vi "pacmate.vi"() -> ()   [LabVIEW 2016]
uses:
  <vilib>/userdefined/High Color/IMAQdx.ctl
  <vilib>/vision/driver/NI_Vision_Acquisition_Software.lvlib
  <vilib>/vision/NI_Vision_Development_Module.lvlib
panel:
  out "filteredDiameter":dbl
  in  "LPF":dbl
  out "Numeric 2":dbl
  out "Numeric":dbl
  out "myDiameter":dbl
  out "Pos. X":i32
  in  "Low Thresh":i32
  in  "Mid Thresh":i32
  out "Min Radius":sgl
  in  "maxThresh":i32
  out "Radius":i32
  in  "Max Radius":sgl=10.0 format="%.2f"
  out "Circles Data":T1(array[cluster])
  out "Nb Circles":i32
  out "Image 3":T2(plugin-control)
  out "Image 2":T2(plugin-control)
  in  "Blue or Luma or Val or Inten Range":cluster{"Lower value":i32, "Upper value":i32}={"Lower value"=0, "Upper value"=255}
  in  "Green or Sat Range":cluster{"Lower value":i32, "Upper value":i32}={"Lower value"=0, "Upper value"=255}
  in  "Red or Hue Range":cluster{"Lower value":i32, "Upper value":i32}={"Lower value"=0, "Upper value"=255}
  out "Image":T2(plugin-control)
  in  "stop":bool
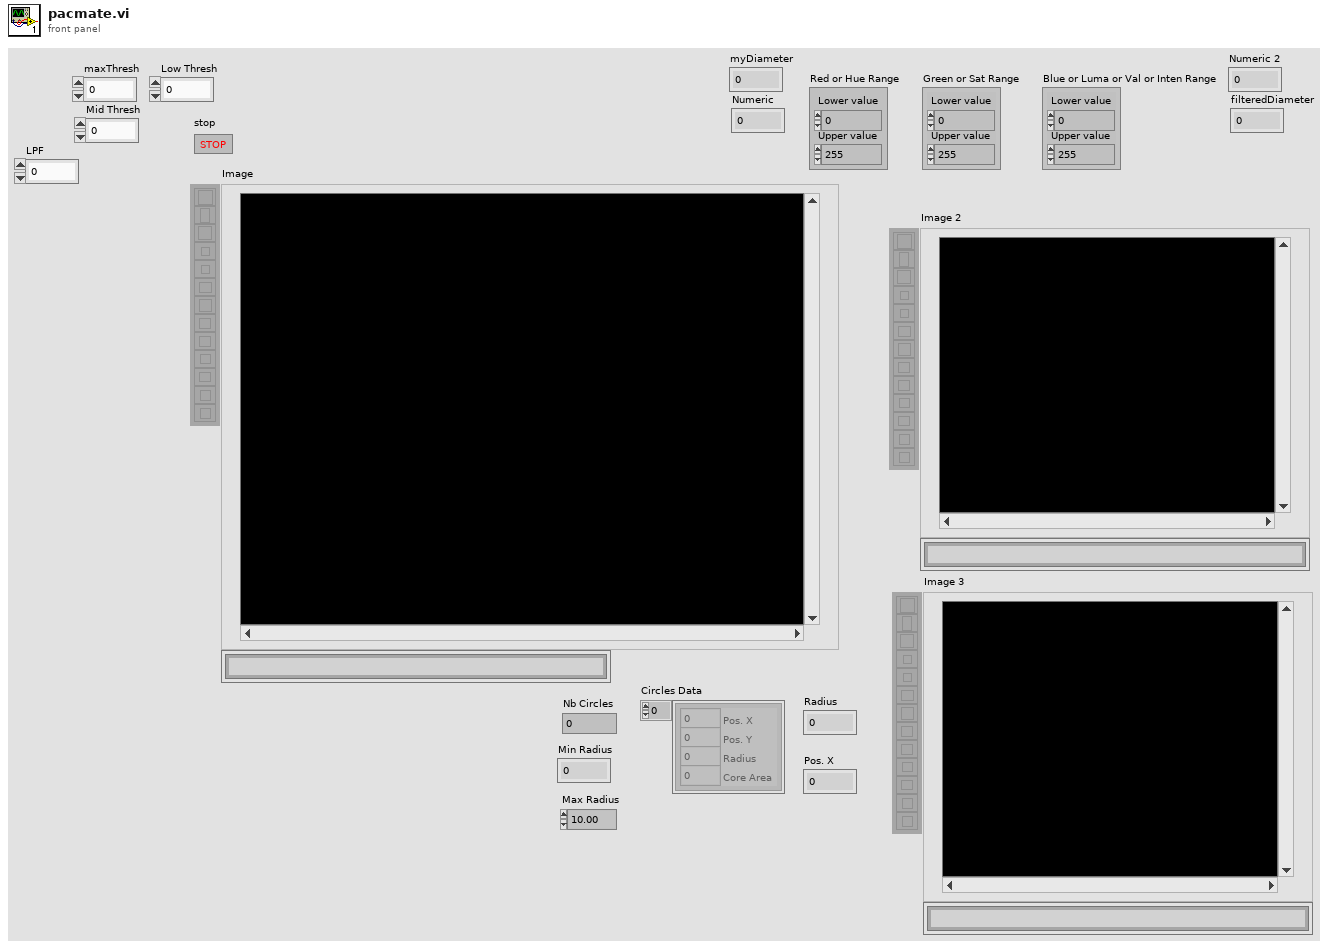
[diagram p1: front panel]
types:
  T1 = cluster{"Pos. X":i32, "Pos. Y":i32, "Radius":i32, "Core Area":i32}[]
  T2 = typedef "IMAQ Image.ctl" = refnum<image>
  T3 = typedef "IMAQdx.ctl" = refnum<k21>
  T4 = cluster{"Pos. X":i32, "Pos. Y":i32, "Radius":i32, "Core Area":i32}
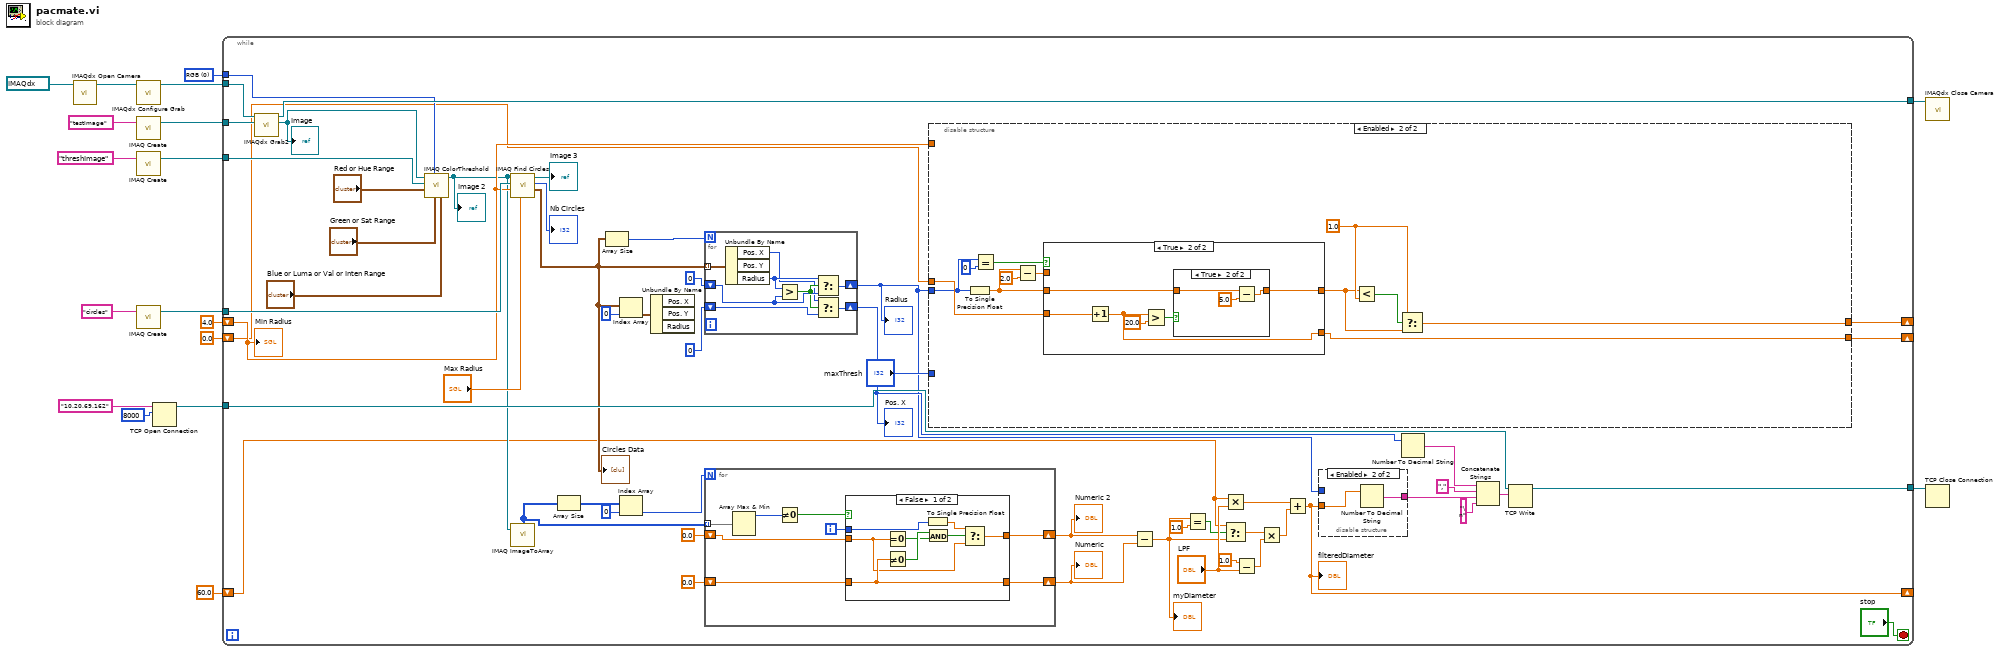
[diagram p0: block diagram]
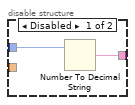
[diagram p2: hidden frame]
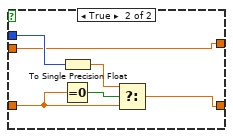
[diagram p3: hidden frame]
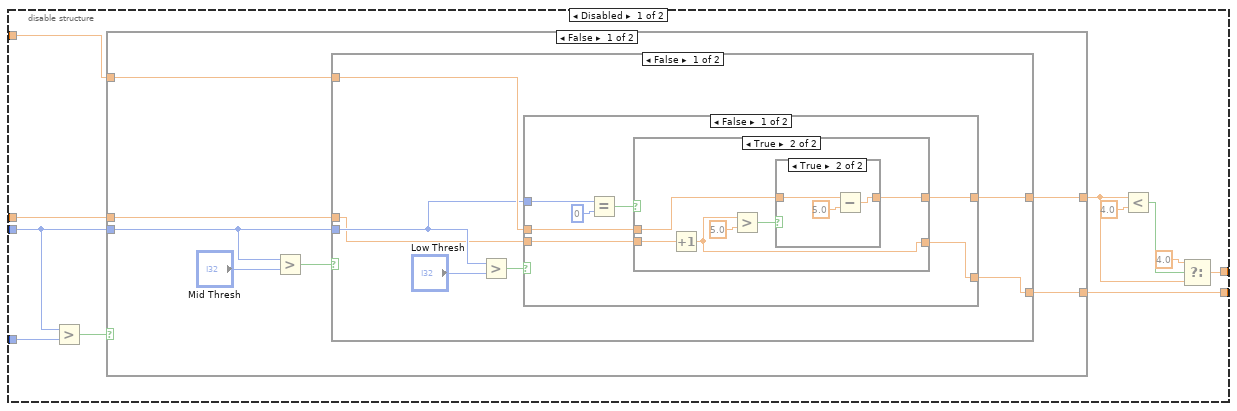
[diagram p4: hidden frame]
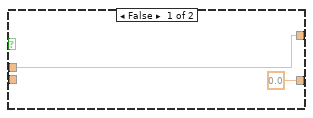
[diagram p5: hidden frame]
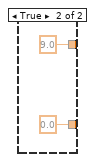
[diagram p7: hidden frame]
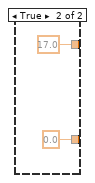
[diagram p8: hidden frame]
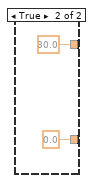
[diagram p9: hidden frame]
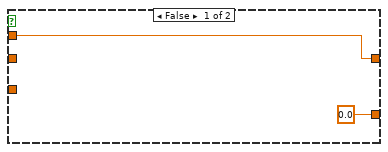
[diagram p10: hidden frame]
diagram:
  w12 = u16 0 items=["RGB", "HSL", "HSV", "HSI"] ("Color Mode")
  n1 = call <vilib>:"IMAQdx Open Camera.vi"("Session In"=T3 "cam1") -> ("Session Out"=w14:T3)  [unwired: 9 in, 1 out]
  n2 = call <vilib>:"IMAQdx Configure Grab.vi"("Session In"=w14) -> ("Session Out"=w13:T3)  [unwired: 9 in, 1 out]
  n3 = call "IMAQ Create"("Image Name"="testImage") -> ("New Image"=w17:T2)  [unwired: 4 in, 1 out]
  n4 = call "IMAQ Create"("Image Name"="threshImage") -> ("New Image"=w10:T2)  [unwired: 4 in, 1 out]
  n5 = call "IMAQ Create"("Image Name"="circles") -> ("New Image"=w8:T2)  [unwired: 4 in, 1 out]
  n6 = TCP Open Connection(address="10.20.69.162", remote port or service name=u16 8000) -> (connection ID=w3:refnum<k5>)  [unwired: 3 in, 1 out]
  n7 = while {
    tunnel: w13 -> [w71]
    tunnel: w17 -> [w70]
    tunnel: [w69] -> w15
    tunnel: w12 -> [w68]
    tunnel: w10 -> [w67]
    tunnel: w8 -> [w63]
    shift-right: [w45] -> _
    shift-left: sgl 4.0 -> [w55]
    shift-right: [w54] -> _
    shift-left: sgl 0.0 -> [w53]
    tunnel: w3 -> [w50]
    tunnel: [w49] -> w2
    shift-right: [w20] -> _
    shift-left: 60.0 -> [w22]
    stop <- "stop" stop-if-true
    n8 = call <vilib>:"IMAQdx Grab2.vi"("Image In"=w70, "Session In"=w71) -> ("Image Out"=w62:T2, "Session Out"=w69:T3)  [unwired: 6 in, 2 out]
    "Image" <- w62
    n9 = call "IMAQ ColorThreshold"("Blue or Luma or Val or Inten Range"="Blue or Luma or Val or Inten Range", "Green or Sat Range"="Green or Sat Range", "Color Mode"=w68, "Red or Hue Range"="Red or Hue Range", "Image Dst"=w67, "Image Src"=w62) -> ("Image Dst Out"=w38:T2)  [unwired: 4 in, 1 out]
    "Image 2" <- w38
    n10 = call "IMAQ Find Circles"("Max Radius"="Max Radius", "Min Radius"=w55, "Image Dst"=w63, "Image Src"=w38) -> ("Circles Data"=w43:T1, "Nb Circles"=→"Nb Circles":i32, "Image Dst Out"=→"Image 3":T2)  [unwired: 4 in, 1 out]
    "Circles Data" <- w43
    n11 = call "IMAQ ImageToArray"("Image"=w38) -> ("Image Pixels (U8)"=w34:u8[][])  [unwired: 3 in, 4 out]
    n12 = Array Size(array=w34) -> (size(s)=w37:i32[])
    n13 = Array Size(array=w43) -> (size(s)=w44:i32)
    n14 = Index Array(array=w43, index=0) -> (element=w57:T4)
    n15 = Index Array(array=w37, index=0) -> (element=w35:i32)
    n16 = Unbundle By Name(w57) -> ()  [unwired: 3 out]
    n17 = for {
      N: w44 -> [_]
      tunnel: w43 -> [w180] mode=indexing
      shift-right: [w178] -> w39
      shift-left: 0 ("y") -> [w177]
      shift-right: [w174] -> w40
      shift-left: 0 ("Pos. X") -> [w173]
      n18 = Unbundle By Name(w180) -> ("Pos. X"=w175:i32, "Radius"=w179:i32)  [unwired: 1 out]
      n19 = Greater?(x=w179, y=w177) -> (0:w176:bool)
      n20 = Select(t=w179, s=w176, f=w177) -> (s? t:f=w178:i32)
      n21 = Select(t=w175, s=w176, f=w173) -> (s? t:f=w174:i32)
    }
    "Radius" <- w39
    "Pos. X" <- w40
    n22 = for {
      N: w35 -> [_]
      tunnel: w34 -> [w84] mode=indexing
      shift-right: [w80] -> w30
      shift-left: 0.0 -> [w79]
      shift-right: [w78] -> w31
      shift-left: 0.0 -> [w77]
      i -> [w81]
      n23 = Array Max & Min(array=w84) -> (max value=w83:u8)  [unwired: 3 out]
      n24 = Not Equal To 0?(x=w83) -> (x != 0?=w82:bool)
      n25 = case shown="False" w82 {
        tunnel: w79 -> [w89 w97]
        tunnel: w81 -> [w92 w96]
        tunnel: [w89 w94] -> w80
        tunnel: w77 -> [w85 w93]
        tunnel: [w90 w93] -> w78
        frame False {
          n26 = Equal To 0?(x=w85) -> (x = 0?=w87:bool)
          n27 = Not Equal To 0?(x=w89) -> (x != 0?=w88:bool)
          n28 = To Single Precision Float(number=w92) -> (single precision float=w91:sgl)
          n29 = And(x=w88, y=w87) -> (x .and. y?=w86:bool)
          n30 = Select(t=w91, s=w86, f=w85) -> (s? t:f=w90:dbl)
        }
        frame True {
          n31 = Equal To 0?(x=w97) -> (x = 0?=w98:bool)
          n32 = To Single Precision Float(number=w96) -> (single precision float=w95:sgl)
          n33 = Select(t=w95, s=w98, f=w97) -> (s? t:f=w94:dbl)
        }
      }
    }
    "Numeric" <- w30
    "Numeric 2" <- w31
    n34 = disable-structure shown="Enabled" {
      disable-tunnel: "maxThresh" -> [w109 _]
      disable-tunnel: w55 -> [w107 _]
      disable-tunnel: [w106 w154] -> w54
      disable-tunnel: w53 -> [w105 w157]
      disable-tunnel: [w100 w149] -> w45
      disable-tunnel: w39 -> [w99 w156]
      frame Disabled {
        n35 = Greater?(x=w99, y=w109) -> (0:w108:bool)
        n36 = case shown="False" w108 {
          tunnel: [w114 sgl 30.0] -> w101
          tunnel: w99 -> [w113 _]
          tunnel: w107 -> [w112 _]
          tunnel: w105 -> [w111 _]
          tunnel: [w110 sgl 0.0] -> w106
          frame False {
            n37 = Greater?(x=w113, y="Mid Thresh") -> (0:w115:bool)
            n38 = case shown="False" w115 {
              tunnel: [w119 sgl 17.0] -> w114
              tunnel: w113 -> [w120 _]
              tunnel: w112 -> [w121 _]
              tunnel: w111 -> [w118 _]
              tunnel: [w117 sgl 0.0] -> w110
              frame False {
                n39 = Greater?(x=w120, y="Low Thresh") -> (0:w122:bool)
                n40 = case shown="False" w122 {
                  tunnel: [w126 sgl 9.0] -> w119
                  tunnel: w121 -> [w127 _]
                  tunnel: w120 -> [w129 _]
                  tunnel: w118 -> [w125 _]
                  tunnel: [w124 sgl 0.0] -> w117
                  frame False {
                    n41 = Equal?(x=w129, y=0) -> (x = y?=w128:bool)
                    n42 = case shown="True" w128 {
                      tunnel: [w132 w133] -> w126
                      tunnel: w127 -> [w132 w134]
                      tunnel: w125 -> [_ w138]
                      tunnel: [sgl 0.0 w137] -> w124
                      frame False {
                      }
                      frame True {
                        n43 = Increment(x=w138) -> (x+1=w137:sgl)
                        n44 = Greater?(x=w137, y=sgl 5.0) -> (0:w135:bool)
                        n45 = case shown="True" w135 {
                          tunnel: w134 -> [w139 w142]
                          tunnel: [w139 w140] -> w133
                          frame False {
                          }
                          frame True {
                            n46 = Subtract(x=w142, y=sgl 5.0) -> (x-y=w140:sgl)
                          }
                        }
                      }
                    }
                  }
                  frame True {
                  }
                }
              }
              frame True {
              }
            }
          }
          frame True {
          }
        }
        n47 = Less?(x=w101, y=4.0) -> (x < y?=w103:bool)
        n48 = Select(t=4.0, s=w103, f=w101) -> (s? t:f=w100:dbl)
      }
      frame Enabled {
        w152 = sgl 1.0 ("y")
        n49 = To Single Precision Float(number=w156) -> (single precision float=w155:sgl)
        n50 = Equal?(x=w156, y=0) -> (x = y?=w159:bool)
        n51 = Subtract(x=w155, y=sgl 2.0) -> (x-y=w153:sgl)
        n52 = case shown="True" w159 {
          tunnel: [w161 w163] -> w150
          tunnel: w155 -> [_ w164]
          tunnel: w157 -> [_ w168]
          tunnel: [sgl 0.0 w167] -> w154
          tunnel: w153 -> [w161 _]
          frame False {
          }
          frame True {
            n53 = Increment(x=w168) -> (x+1=w167:sgl)
            n54 = Greater?(x=w167, y=sgl 20.0) -> (0:w165:bool)
            n55 = case shown="True" w165 {
              tunnel: w164 -> [w169 w172]
              tunnel: [w169 w170] -> w163
              frame False {
              }
              frame True {
                n56 = Subtract(x=w172, y=sgl 5.0) -> (x-y=w170:sgl)
              }
            }
          }
        }
        n57 = Less?(x=w150, y=w152) -> (x < y?=w151:bool)
        n58 = Select(t=w152, s=w151, f=w150) -> (s? t:f=w149:sgl)
      }
    }
    n59 = Subtract(x=w31, y=w30) -> (x-y=w19:dbl)
    "myDiameter" <- w19
    n60 = Equal?(x=w19, y=1.0) -> (x = y?=w23:bool)
    n61 = Multiply(x=w22, y="LPF") -> (x*y=w26:dbl)
    n62 = Select(t=w22, s=w23, f=w19) -> (s? t:f=w21:dbl)
    n63 = Subtract(x=1.0, y="LPF") -> (x-y=w27:dbl)
    n64 = Multiply(x=w21, y=w27) -> (x*y=w25:dbl)
    n65 = Add(x=w26, y=w25) -> (x+y=w20:dbl)
    "filteredDiameter" <- w20
    n66 = disable-structure shown="Enabled" {
      disable-tunnel: [w74 w75] -> w48
      disable-tunnel: w39 -> [w73 _]
      disable-tunnel: w20 -> [_ w76]
      frame Disabled {
        n67 = Number To Decimal String(number=w73) -> (decimal integer string=w74:string)  [unwired: 1 in]
      }
      frame Enabled {
        n68 = Number To Decimal String(number=w76) -> (decimal integer string=w75:string)  [unwired: 1 in]
      }
    }
    n69 = Number To Decimal String(number=w40) -> (decimal integer string=w52:string)  [unwired: 1 in]
    n70 = Concatenate Strings(w52, "," ("string"), w48, "\n" ("string")) -> (w51:string)
    n71 = TCP Write(connection ID=w50, data in=w51) -> (connection ID out=w49:refnum<k5>)  [unwired: 2 in, 2 out]
    "Min Radius" <- w55
  }
  n72 = call <vilib>:"IMAQdx Close Camera.vi"("Session In"=w15) -> ()  [unwired: 10 in, 1 out]
  n73 = TCP Close Connection(connection ID=w2) -> ()  [unwired: 2 in, 2 out]
